vi "CHROMA Clear Output Protection.vi"(8 "Error In":errorcluster, 11 "CHROMA VISA In":refnum<visa-resource-name>) -> (0 "Error Out":errorcluster, 2 "Instrument Name":string, 3 "CHROMA VISA Out":refnum<visa-resource-name>)   [LabVIEW 2018]
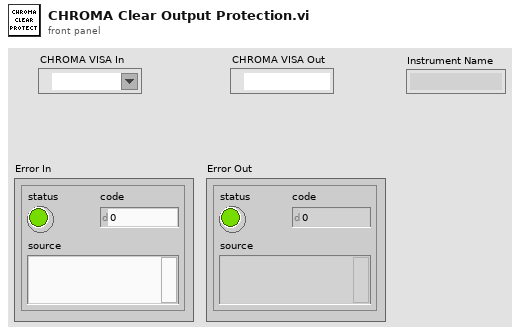
[diagram p1: front panel]
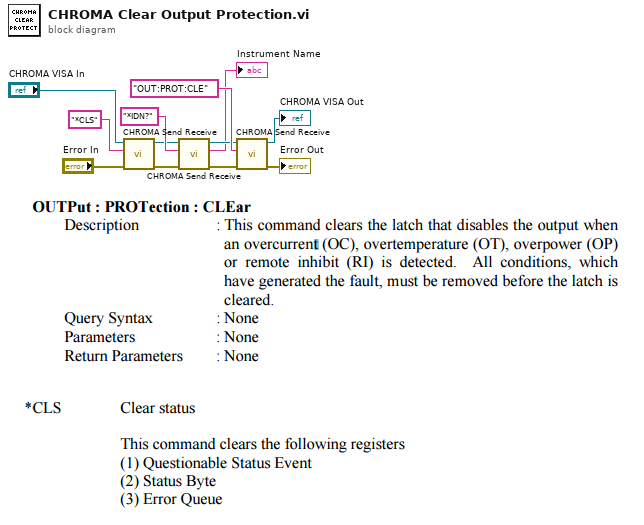
[diagram p0: block diagram]
diagram:
  n1 = call "CHROMA Send Receive.vi"("error in (no error)"="Error In", "Send Command"="*CLS" ("string to write"), "CHROMA VISA In"="CHROMA VISA In") -> ("error out"=w5:errorcluster, "CHROMA VISA Out"=w3:refnum<visa-resource-name>)  [unwired: 6 in, 1 out]
  n2 = call "CHROMA Send Receive.vi"("error in (no error)"=w5, "Send Command"="*IDN?", "CHROMA VISA In"=w3) -> ("error out"=w4:errorcluster, "read buffer"=→"Instrument Name":string, "CHROMA VISA Out"=w2:refnum<visa-resource-name>)  [unwired: 6 in]
  n3 = call "CHROMA Send Receive.vi"("error in (no error)"=w4, "Send Command"="OUT:PROT:CLE" ("string to write"), "CHROMA VISA In"=w2) -> ("error out"=→"Error Out":errorcluster, "CHROMA VISA Out"=→"CHROMA VISA Out":refnum<visa-resource-name>)  [unwired: 6 in, 1 out]
